vi "gfitsio-get-column-name.vi"(8 "error in (no error)":errorcluster, 10 "column number":i32, 11 "Refnum in":T1) -> (0 "error out":errorcluster, 2 "column name":string, 3 "Refnum out":T1)   [LabVIEW 2023, in "gfitsio.lvlib"]
uses:
  gfitsio.lvlib
  gfitsio-refnum.ctl
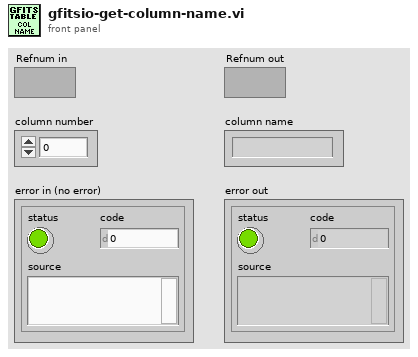
[diagram p1: front panel]
types:
  T1 = typedef "gfitsio.lvlib/gfitsio-refnum.ctl" = refnum<k1>
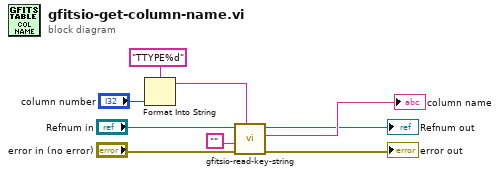
[diagram p0: block diagram]
diagram:
  n1 = Format Into String(format string="TTYPE%d", "column number") -> (resulting string=w5:string)  [unwired: 2 in, 1 out]
  n2 = call "gfitsio-read-key-string.vi"("keyname"=w5, "error in (no error)"="error in (no error)", "default value"="", "gfits refnum"="Refnum in") -> ("error out"=→"error out":errorcluster, "value"=→"column name":string, "dup gfits refnum"=→"Refnum out":T1)  [unwired: 4 in, 1 out]
